vi "Get Event Case Terminals For RPC VI connection.vi"(10 "Event  Inner Case Termianls":refnum<vi>[](array[refnum])) -> (0 "error out Term":refnum<vi>, 1 "error in Term":refnum<vi>, 2 "Service out Term":refnum<vi>, 3 "Service in Term":refnum<vi>)   [LabVIEW 2019, in "gRPC Template Creation Utility.lvlib"]
uses:
  gRPC Template Creation Utility.lvlib
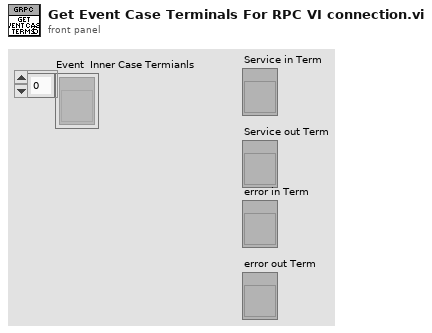
[diagram p1: front panel]
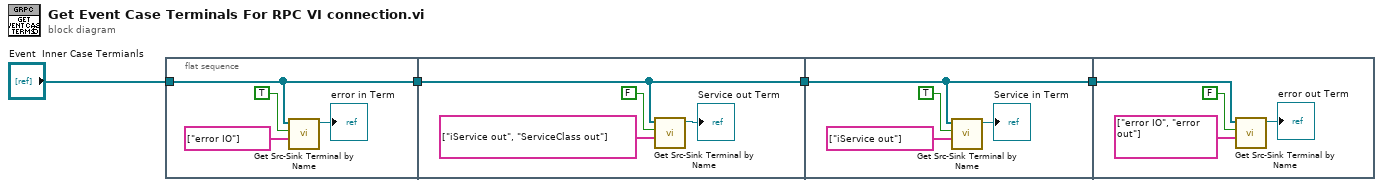
[diagram p0: block diagram]
diagram:
  n1 = flat-sequence {
    tunnel: "Event  Inner Case Termianls" -> [w6]
    tunnel: [w6] -> w3
    tunnel: w3 -> [w10]
    tunnel: [w10] -> w2
    tunnel: w2 -> [w14]
    tunnel: [w14] -> w1
    tunnel: w1 -> [w18]
    frame #0 {
      n2 = call "Get Src-Sink Terminal by Name.vi"("Poosible Terminal Names"=string[] ["error IO"], "Find Source"=TRUE, "Event Case Termianls"=w6) -> ("Term Refnum out"=→"error in Term":refnum<vi>)  [unwired: 8 in]
    }
    frame #1 {
      n3 = call "Get Src-Sink Terminal by Name.vi"("Poosible Terminal Names"=string[] ["iService out", "ServiceClass out"], "Find Source"=FALSE, "Event Case Termianls"=w10) -> ("Term Refnum out"=→"Service out Term":refnum<vi>)  [unwired: 8 in]
    }
    frame #2 {
      n4 = call "Get Src-Sink Terminal by Name.vi"("Poosible Terminal Names"=string[] ["iService out"], "Find Source"=TRUE, "Event Case Termianls"=w14) -> ("Term Refnum out"=→"Service in Term":refnum<vi>)  [unwired: 8 in]
    }
    frame #3 {
      n5 = call "Get Src-Sink Terminal by Name.vi"("Poosible Terminal Names"=string[] ["error IO", "error out"], "Find Source"=FALSE, "Event Case Termianls"=w18) -> ("Term Refnum out"=→"error out Term":refnum<vi>)  [unwired: 8 in]
    }
  }
